vi "CCExcelToDcm.vi"(6 "DICOM Info":path, 8 "error in (no error)":errorcluster, 10 "JournalPath":path, 11 "ServerInfo":T1) -> (0 "error out":errorcluster, 1 "No active excel error":bool, 2 "VerificationFailure":string, 3 "FailureDescription":string)   [LabVIEW 2013, in "main.lvlib" / "ClearCanvasLibrary.lvlib"]
uses:
  ClearCanvasLibrary.lvlib
  C:/Users/Simon/SkyDrive/LabView/2013/DM2020/DICOM/ClearCanvasNewBuild/ClearCanvas.Dicom.dll
  ClearCanvasNewBuild/ClearCanvas.Dicom.dll
  <userlib>/_MGI/Error Handling/MGI Suppress Error Code/MGI Suppress Error Code (Scalar).vi
  main.lvlib
  Controls/Enum Variables.ctl
panel:
  in  "Excel._Worksheet":refnum<k7>
  in  "Excel._Application":refnum<k7>
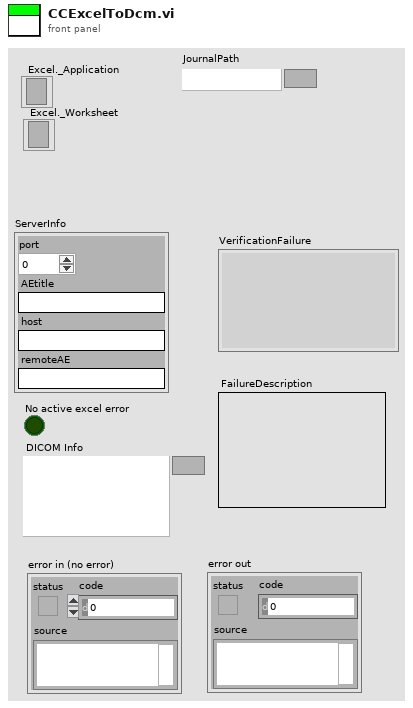
[diagram p1: front panel]
types:
  T1 = cluster{"port":i32, "AEtitle":string, "host":string, "remoteAE":string}
  T2 = typedef "main.lvlib/Enum Variables.ctl" = enum16{"SetAcqFilter", "GetAcqFilter", "Set Filter", "Get Filter", "Set Height", "Get Height", "Set Blue Pressure", "Get Blue Pressure", "Set Red Pressure", "Get Red Pressure", "Init", "Reset Pressure", "Set Red Cursors", "Get Red Cursors", "Set Blue Cursors", "Get Blue Cursors", "Set Language", "Get Language", "Set Active Graphs", "Get ActiveGraphs", "Set Method", "Get Method", "Set Encryption", "Get Encryption", "Set ExcelVersion", "Get ExcelVersion", "Set DICOM Avail", "Get DICOM Avail", "Set DICOM Encode", "Get DICOM Encode", "Set JournalExport", "Get JournalExport", "Set Sequence", "Get Sequence", "Set DAQ Connected", "Get DAQ Connected", "Set Current Graph", "Get Current Graph", "Set General Settings", "Get Hyphenation", "Set Arm Calc Method", "Get Arm Calc Method", "Set Dicom Tags", "Get Dicom Tags", "Set BT Serial", "Get BT Serial", "Set BT Accepted Serials", "Get BT Accepted Serials", "Get BT License", "Set BT License"}
  T3 = enum16{"leave excel open after last close", "close only if opened by LabVIEW", "close excel after last close"}
  T4 = enum16{"open workbook as template", "open workbook from file", "create new workbook"}
  T5 = typedef "excel Object Reference.ctl" = refnum<k1>
  T6 = typedef "excel Data Members.ctl" = cluster{"Excel._Application":refnum<k7>, "Excel._Workbook":refnum<k7>, "Excel._Worksheet":refnum<k7>, "template?":bool, "location":cluster{"TopLeft":string, "RightBottom":string}, "positioning info":cluster{"direction":enum16{"right", "down"}, "gap":i32}}
  T7 = cluster{"left":i16, "top":i16, "right":i16, "bottom":i16}
  T8 = cluster{"left":i32, "top":i32, "right":i32, "bottom":i32}
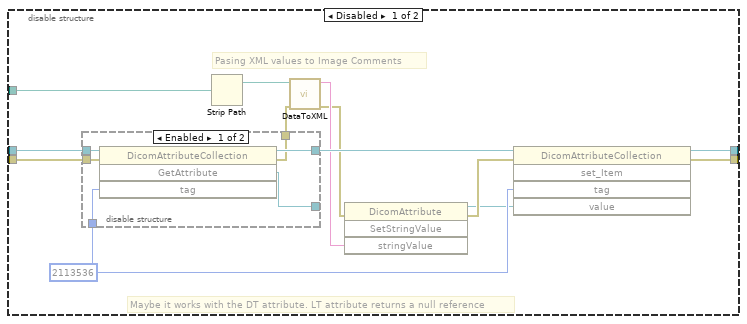
[diagram p2: hidden frame]
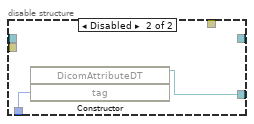
[diagram p3: hidden frame]
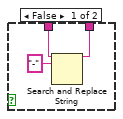
[diagram p4: hidden frame]
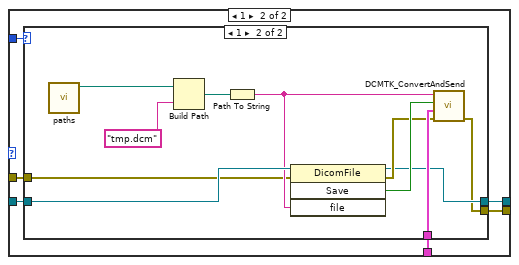
[diagram p5: hidden frame]
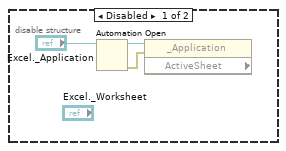
[diagram p7: hidden frame]
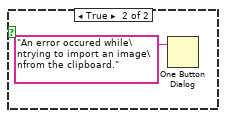
[diagram p8: hidden frame]
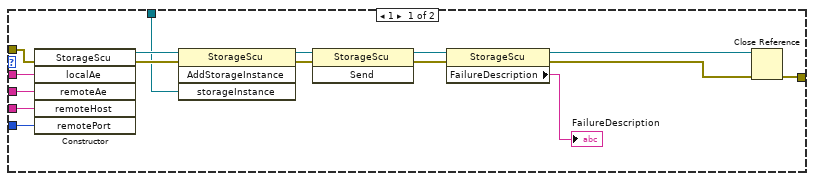
[diagram p9: hidden frame]
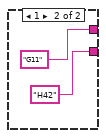
[diagram p11: hidden frame]
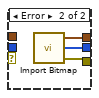
[diagram p12: hidden frame]
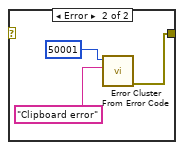
[diagram p13: hidden frame]
diagram:
  w67 = 6 items=["None", "CR", "CT", "MR", "NM", "US", "OT", "BI", "CD", "DD", "DG", "ES", "LS", "PT", "RG", "ST", "TG", "XA", "RF", "RTImage", "RTDose", "RTStruct", "RTPlan", "RTRecord", "HC", "DX", "MG", "IO", "PX", "GM", "SM", "XC", "PR", "AU", "Ecg", "Eps", "HD", "SR", "Ivus", "OP", "Smr", "Oct", "Opr", "Opv", "Opm", "KO", "Seg", "Reg", "DS", "CF", "DF", "VF", "AS", "CS", "EC", "LP", "FA", "CP", "DM", "FS", "MA", "MS"] ("Modality")
  n1 = disable-structure shown="Enabled" {
    frame Disabled {
      n2 = Automation Open(Automation Refnum="Excel._Application") -> (Automation Refnum=w150:refnum<k7>, error out=w149:errorcluster)  [unwired: 3 in]
      n3 = property class="_Application" props=["ActiveSheet"](reference=w150, error in=w149) -> ()  [unwired: 3 out]
    }
    frame Enabled {
    }
  }
  n4 = call <userlib>:"excel open (path).vi"("Visible (T)"=FALSE, "closing behavior (leave open)"=T3."close excel after last close", "worksheet_number"=u8 2, "workbook path"="JournalPath", "error in (no error)"="error in (no error)", "select/new"=enum16{"new sheet", "select sheet"}."select sheet", "create/open template/open file"=T4."open workbook from file") -> ("error out"=w31:errorcluster, "reference"=w32:T5)  [unwired: 3 in]
  n5 = call <userlib>:"excel Get Data to Modify.vi"("error in (no error)"=w31, "reference"=w32) -> ("error out"=w29:errorcluster, "data"=w23:T6, "duplicate reference"=w25:T5)  [unwired: 2 in, 1 out]
  n6 = Unbundle By Name(w23) -> ("Excel._Worksheet"=w30:refnum<k7>)
  n7 = while {
    tunnel: w29 -> [w165]
    tunnel: [w164] -> w96
    tunnel: [w159] -> w88
    tunnel: [w163] -> w92
    tunnel: [w160] -> w89
    tunnel: w30 -> [w155]
    stop <- w156 stop-if-true
    w169 = 2 items=["xlBitmap"=2, "xlPicture"=-4147] ("Format")
    w170 = 1 items=["xlPrinter"=2, "xlScreen"=1] ("Appearance")
    n8 = call "AE Variables.vi"("Action"=Enum_Variables."Get JournalExport") -> ("RingOut"=w152:u16)  [unwired: 11 in, 7 out]
    n9 = case shown="0, Default" w152 {
      tunnel: ["A1" "G11"] -> w168
      tunnel: ["H49" "H42"] -> w167
      frame 0, Default {
      }
      frame 1 {
      }
    }
    n10 = invoke class="_Worksheet" method="Range"(reference=w155, error in=w165, "Cell1"=w168, "Cell2"=w167) -> (error out=w166:errorcluster, "Range"=w171:refnum<k7>)  [unwired: 1 in, 3 out]
    n11 = invoke class="Range" method="CopyPicture"(reference=w171, error in=w166, "Appearance"=w170, "Format"=w169) -> (reference out=w160:refnum<k7>, error out=w154:errorcluster)  [unwired: 1 in, 3 out]
    n12 = case shown="No Error" w154 {
      selector: w154 -> [w176 w194]
      tunnel: [w182 _] -> w164
      tunnel: [w183 _] -> w163
      tunnel: [w180 w194] -> w159
      frame No Error {
        n13 = call "ImportBitmap2.vi"("error in (no error)"=w176) -> ("error out"=w177:errorcluster, "pixmap data"=w178:u8[], "rect"=w179:T7)  [unwired: 6 in, 2 out]
        n14 = case shown="No Error" w177 {
          selector: w177 -> [w184 _]
          tunnel: [w186 w189] -> w183
          tunnel: w179 -> [w186 _]
          tunnel: w178 -> [w185 _]
          tunnel: [w185 w188] -> w182
          tunnel: [w184 w187] -> w181
          frame No Error {
          }
          frame Error {
            n15 = call "Import Bitmap.vi"() -> ("rect"=w189:T8, "flattened data"=w188:u8[], "error out"=w187:errorcluster)  [unwired: 5 in, 2 out]
          }
        }
        n16 = case shown="No Error" w181 {
          selector: w181 -> [w190 _]
          tunnel: [w190 w193] -> w180
          frame No Error {
          }
          frame Error {
            n17 = call <vilib>:"Error Cluster From Error Code.vi"("error message (\"\")"="Clipboard error" ("error message (\"\")"), "error code (0)"=50001) -> ("error out"=w193:errorcluster)  [unwired: 7 in]
          }
        }
      }
      frame Error {
      }
    }
    n18 = Unbundle By Name(w159) -> ("status"=w157:bool)
    n19 = Unbundle By Name(w163) -> ("bottom"=w162:i32)
    n20 = Less?(x=500, y=w162) -> (x < y?=w158:bool)
    n21 = Or(x=w158, y=w157) -> (x .or. y?=w156:bool)
  }
  n22 = Close Reference(reference=w89, error in (no error)=w88) -> (error out=w28:errorcluster)
  n23 = Path To String(path="DICOM Info") -> (string=w18:string)
  n24 = call <userlib>:"excel Set Modified Data.vi"("error in (no error)"=w28, "data"=w23, "reference"=w25) -> ("error out"=w27:errorcluster, "duplicate reference"=w24:T5)  [unwired: 3 in]
  n25 = call <userlib>:"excel close.vi"("error in (no error)"=w27, "reference"=w24) -> ("error out"=w26:errorcluster)  [unwired: 9 in]
  n26 = invoke class="DicomUid" method="GenerateUid"(error in=w26) -> (error out=w147:errorcluster, "GenerateUid"=w102:refnum<k24>)  [unwired: 2 in, 1 out]
  n27 = constructor class="DicomTagDictionary"(error in=w26) -> (reference out=w141:refnum<k24>, error out=w137:errorcluster)  [unwired: 2 in, 1 out]
  n28 = constructor class="DicomFile"(error in=w26, "filename"=w18) -> (reference out=w101:refnum<k24>, error out=w100:errorcluster)  [unwired: 2 in, 2 out]
  n29 = invoke class="DicomFile" method="Load"(reference=w101, error in=w100) -> (reference out=w55:refnum<k24>, error out=w99:errorcluster)  [unwired: 1 in, 1 out]
  n30 = property class="DicomUid"(reference=w102, error in=w147) -> (reference out=w93:refnum<k24>, error out=w94:errorcluster, "UID"=w138:string)
  n31 = property class="DicomFile"(reference=w55, error in=w99, "MediaStorageSopClassUid"="1.2.840.10008.5.1.4.1.1.7" ("uid"), "MediaStorageSopInstanceUid"=w138, "TransferSyntaxUid"="1.2.840.10008.1.2.1") -> (reference out=w144:refnum<k24>, error out=w143:errorcluster)
  n32 = Close Reference(reference=w93, error in (no error)=w94) -> (error out=w9:errorcluster)
  n33 = invoke class="DicomTagDictionary" method="GetDicomTag"(reference=w141, error in=w137, "name"="SopInstanceUid") -> (reference out=w17:refnum<k24>, error out=w16:errorcluster, "GetDicomTag"=w139:refnum<k24>)  [unwired: 1 in, 1 out]
  n34 = property class="DicomFile"(reference=w144, error in=w143) -> (reference out=w54:refnum<k24>, error out=w107:errorcluster, "DataSet"=w142:refnum<k24>)
  n35 = constructor class="DicomAttributeUI"(error in=w107, "tag"=w139) -> (reference out=w130:refnum<k24>, error out=w132:errorcluster)  [unwired: 2 in, 2 out]
  n36 = invoke class="DicomAttributeUI" method="SetStringValue"(reference=w130, error in=w132, "stringValue"=w138) -> (reference out=w131:refnum<k24>, error out=w106:errorcluster)  [unwired: 1 in, 2 out]
  n37 = invoke class="DicomAttributeCollection" method="set_Item"(reference=w142, error in=w106, "tag"=w139, "value"=w131) -> (reference out=w2:refnum<k24>, error out=w1:errorcluster)  [unwired: 1 in, 3 out]
  n38 = disable-structure shown="Enabled" {
    disable-tunnel: "DICOM Info" -> [w207 _]
    disable-tunnel: [w206 w219] -> w11
    disable-tunnel: [w205 w218] -> w8
    disable-tunnel: w2 -> [w196 w219]
    disable-tunnel: w1 -> [w195 w218]
    frame Disabled {
      w204 = u32 2113536 ("tag")
      # "Pasing XML values to Image Comments"
      # "Maybe it works with the DT attribute. LT attribute returns a null reference"
      n39 = disable-structure shown="Enabled" {
        disable-tunnel: [w213 w216] -> w202
        disable-tunnel: [w212 w215] -> _
        disable-tunnel: [w211 w217] -> w198
        disable-tunnel: w204 -> [w210 w214]
        disable-tunnel: w196 -> [w209 _]
        disable-tunnel: w195 -> [w208 _]
        frame Enabled {
          n40 = invoke class="DicomAttributeCollection" method="GetAttribute"(reference=w209, error in=w208, "tag"=w210) -> (reference out=w213:refnum<k24>, error out=w211:errorcluster, "GetAttribute"=w212:refnum<k24>)  [unwired: 1 in, 1 out]
        }
        frame Disabled {
          n41 = constructor class="DicomAttributeDT"("tag"=w214) -> (reference out=w215:refnum<k24>)  [unwired: 3 in, 3 out]
        }
      }
      n42 = Strip Path(path=w207) -> (stripped path=w203:path)  [unwired: 1 out]
      n43 = call "DataToXML.vi"("error in"=w198, "path"=w203) -> ("error out"=w197:errorcluster, "XML"=w199:string)  [unwired: 8 in]
      n44 = invoke class="DicomAttribute" method="SetStringValue"(error in=w197, "stringValue"=w199) -> (reference out=w200:refnum<k24>, error out=w201:errorcluster)  [unwired: 2 in, 2 out]
      n45 = invoke class="DicomAttributeCollection" method="set_Item"(reference=w202, error in=w201, "tag"=w204, "value"=w200) -> (reference out=w206:refnum<k24>, error out=w205:errorcluster)  [unwired: 1 in, 3 out]
    }
    frame Enabled {
    }
  }
  n46 = invoke class="DicomTagDictionary" method="GetDicomTag"(reference=w17, error in=w16, "name"="SopClassUid") -> (reference out=w58:refnum<k24>, error out=w57:errorcluster, "GetDicomTag"=w109:refnum<k24>)  [unwired: 1 in, 1 out]
  n47 = Close Reference(reference=w58, error in (no error)=w57) -> (error out=w56:errorcluster)
  n48 = call "CCSetSpecificCharacterSet.vi"("error in (no error)"=w8, ".NET Refnum in"=w11) -> ("error out"=w7:errorcluster, ".NET Refnum out"=w10:refnum<k24>)  [unwired: 8 in]
  n49 = property class="SopClass"(error in=w56) -> (reference out=w61:refnum<k24>, error out=w60:errorcluster, "SecondaryCaptureImageStorageUid"=w111:string)  [unwired: 1 in]
  n50 = constructor class="DicomAttributeUI"(error in=w7, "tag"=w109) -> (reference out=w113:refnum<k24>, error out=w112:errorcluster)  [unwired: 2 in, 2 out]
  n51 = invoke class="DicomAttributeUI" method="SetStringValue"(reference=w113, error in=w112, "stringValue"=w111) -> (reference out=w110:refnum<k24>, error out=w108:errorcluster)  [unwired: 1 in, 2 out]
  n52 = Close Reference(reference=w61, error in (no error)=w60) -> (error out=w59:errorcluster)
  n53 = invoke class="DicomAttributeCollection" method="set_Item"(reference=w10, error in=w108, "tag"=w109, "value"=w110) -> (reference out=w5:refnum<k24>, error out=w91:errorcluster)  [unwired: 1 in, 3 out]
  n54 = Merge Errors(w91, w9, w59) -> (w90:errorcluster)
  n55 = constructor class="PatientModuleIod"(error in=w90, "dicomAttributeProvider"=w5) -> (reference out=w98:refnum<k24>, error out=w97:errorcluster)  [unwired: 2 in, 2 out]
  n56 = property class="PatientModuleIod"(reference=w98, error in=w97) -> (reference out=w73:refnum<k24>, error out=w72:errorcluster, "PatientsName"=w69:string, "PatientId"=w15:string)
  n57 = call "AE Variables.vi"("Action"=Enum_Variables."Get Hyphenation") -> ("BooleanOut"=w12:bool)  [unwired: 11 in, 7 out]
  n58 = case shown="True" w12 {
    tunnel: w15 -> [w222 w223]
    tunnel: [w220 w223] -> w14
    frame False {
      n59 = Search and Replace String(input string=w222, search string="-") -> (result string=w220:string)  [unwired: 6 in, 3 out]
    }
    frame True {
    }
  }
  n60 = call "NameToDICOMFormat.vi"("Name In"=w69) -> ("Name Out"=w68:string)  [unwired: 10 in]
  n61 = property class="PatientModuleIod"(reference=w73, error in=w72, "PatientsName"=w68, "PatientId"=w14) -> (reference out=w70:refnum<k24>, error out=w71:errorcluster)
  n62 = Close Reference(reference=w70, error in (no error)=w71) -> (error out=w127:errorcluster)
  n63 = constructor class="GeneralStudyModuleIod"(error in=w127, "dicomAttributeProvider"=w5) -> (reference out=w86:refnum<k24>, error out=w87:errorcluster)  [unwired: 2 in, 2 out]
  n64 = property class="GeneralStudyModuleIod"(reference=w86, error in=w87) -> (reference out=w85:refnum<k24>, error out=w84:errorcluster, "StudyInstanceUid"=w83:string, "ReferringPhysiciansName"=w75:string)
  n65 = call "CCExcelToDcmGenerateUIDs.vi"("String in"=w83) -> ("String out"=w82:string)  [unwired: 10 in]
  n66 = call "NameToDICOMFormat.vi"("Name In"=w75) -> ("Name Out"=w74:string)  [unwired: 10 in]
  n67 = property class="GeneralStudyModuleIod"(reference=w85, error in=w84, "StudyInstanceUid"=w82, "ReferringPhysiciansName"=w74) -> (reference out=w136:refnum<k24>, error out=w135:errorcluster)
  n68 = Close Reference(reference=w136, error in (no error)=w135) -> (error out=w129:errorcluster)
  n69 = constructor class="GeneralSeriesModuleIod"(error in=w129, "provider"=w5) -> (reference out=w81:refnum<k24>, error out=w80:errorcluster)  [unwired: 2 in, 2 out]
  n70 = property class="GeneralSeriesModuleIod"(reference=w81, error in=w80) -> (reference out=w79:refnum<k24>, error out=w78:errorcluster, "SeriesInstanceUid"=w77:string, "OperatorsName"=w66:string)
  n71 = call "NameToDICOMFormat.vi"("Name In"=w66) -> ("Name Out"=w65:string)  [unwired: 10 in]
  n72 = call "CCExcelToDcmGenerateUIDs.vi"("String in"=w77) -> ("String out"=w76:string)  [unwired: 10 in]
  n73 = property class="GeneralSeriesModuleIod"(reference=w79, error in=w78, "SeriesInstanceUid"=w76, "OperatorsName"=w65, "Modality"=w67) -> (reference out=w134:refnum<k24>, error out=w133:errorcluster)
  n74 = Close Reference(reference=w134, error in (no error)=w133) -> (error out=w128:errorcluster)
  n75 = constructor class="ImagePixelMacroIod"(error in=w128, "dicomAttributeProvider"=w5) -> (reference out=w126:refnum<k24>, error out=w64:errorcluster)  [unwired: 2 in, 2 out]
  n76 = property class="PhotometricInterpretation"(error in=w64) -> (error out=w63:errorcluster, "Rgb"=w115:refnum<k24>)  [unwired: 1 in, 1 out]
  n77 = invoke class="ImagePixelMacroIod" method="SetCommonTags"(reference=w126, error in=w63) -> (reference out=w125:refnum<k24>, error out=w124:errorcluster)  [unwired: 1 in, 1 out]
  n78 = Unbundle By Name(w92) -> ("right"=w117:i32, "bottom"=w116:i32)
  n79 = property class="ImagePixelMacroIod"(reference=w125, error in=w124, "BitsAllocated"=u16 8, "BitsStored"=u16 8, "HighBit"=u16 7, "PixelRepresentation"="0", "PlanarConfiguration"=u16 0, "SamplesPerPixel"=u16 3, "PixelData"=w96, "Columns"=w117, "Rows"=w116, "PhotometricInterpretation"=w115) -> (reference out=w62:refnum<k24>, error out=w95:errorcluster)
  n80 = Close Reference(reference=w62, error in (no error)=w95) -> (error out=w6:errorcluster)
  n81 = call "CCSetSpecificCharacterSet.vi"("error in (no error)"=w6, ".NET Refnum in"=w5) -> ("error out"=w3:errorcluster, ".NET Refnum out"=w4:refnum<k24>)  [unwired: 8 in]
  n82 = Close Reference(reference=w4, error in (no error)=w3) -> (error out=w48:errorcluster)
  n83 = Unbundle By Name("ServerInfo") -> ("AEtitle"=w45:string, "remoteAE"=w42:string, "host"=w43:string, "port"=w44:i32)
  n84 = call "CCVerificationSCU.vi"("remotePort"=w44, "error in (no error)"=w48, "remoteHost"=w43, "remoteAE"=w42, "clientAETitle"=w45) -> ("error out"=w47:errorcluster, "FailureDescription"=→"VerificationFailure":string, "Result"=w20:i32)  [unwired: 4 in]
  n85 = call "AE Variables.vi"("Action"=Enum_Variables."Get DICOM Encode") -> ("RingOut"=w51:u16)  [unwired: 11 in, 7 out]
  n86 = case shown="0, Default" w20 {
    tunnel: w54 -> [w224 w233]
    tunnel: [w224 w232] -> w53
    tunnel: w51 -> [_ w231]
    tunnel: [w225 w230] -> w50
    tunnel: w47 -> [w226 w229]
    tunnel: "ServerInfo" -> [_ w228]
    frame 0, Default {
      n87 = call <vilib>:"Error Cluster From Error Code.vi"("error in (no error)"=w226, "error code (0)"=51000) -> ("error out"=w225:errorcluster)  [unwired: 7 in]
    }
    frame 1 {
      n88 = case shown="1" w231 {
        tunnel: w233 -> [w235 w243]
        tunnel: w228 -> [_ w240]
        tunnel: w229 -> [w234 w239]
        tunnel: [w235 w237] -> w232
        tunnel: [w234 w236] -> w230
        frame 0, Default {
        }
        frame 1 {
          n89 = call "paths.vi"() -> ("PubAppData"=w246:path)  [unwired: 8 in, 3 out]
          n90 = Build Path(base path=w246, name or relative path="tmp.dcm") -> (appended path=w244:path)
          n91 = Path To String(path=w244) -> (string=w242:string)
          n92 = invoke class="DicomFile" method="Save"(reference=w243, error in=w239, "file"=w242) -> (reference out=w237:refnum<k24>, error out=w238:errorcluster, "Save"=w241:bool)  [unwired: 1 in, 1 out]
          n93 = call "DCMTK_ConvertAndSend.vi"("error in (no error)"=w238, "ServerInfo"=w240, "Saved?"=w241, "File Input"=w242) -> ("error out"=w236:errorcluster)  [unwired: 6 in, 1 out]
        }
      }
    }
  }
  n94 = case shown="0, Default" w51 {
    tunnel: [w257 w277] -> w146
    tunnel: w50 -> [w256 w277]
    tunnel: w53 -> [w255 _]
    tunnel: w45 -> [w251 _]
    tunnel: w42 -> [w250 _]
    tunnel: w43 -> [w249 _]
    tunnel: w44 -> [w248 _]
    tunnel: w20 -> [w247 _]
    frame 0, Default {
      n95 = constructor class="StorageInstance"(error in=w256, "dicomFile"=w255) -> (reference out=w254:refnum<k24>, error out=w252:errorcluster)  [unwired: 2 in, 2 out]
      n96 = case shown="0, Default" w247 {
        tunnel: [w265 w274] -> w253
        tunnel: w254 -> [w268 _]
        tunnel: w252 -> [w262 w275]
        tunnel: w251 -> [w261 _]
        tunnel: w250 -> [w260 _]
        tunnel: w249 -> [w259 _]
        tunnel: w248 -> [w258 _]
        frame 1 {
          n97 = constructor class="StorageScu"(error in=w262, "localAe"=w261, "remoteAe"=w260, "remoteHost"=w259, "remotePort"=w258) -> (reference out=w270:refnum<k24>, error out=w269:errorcluster)  [unwired: 2 in, 5 out]
          n98 = invoke class="StorageScu" method="AddStorageInstance"(reference=w270, error in=w269, "storageInstance"=w268) -> (reference out=w272:refnum<k24>, error out=w271:errorcluster)  [unwired: 1 in, 2 out]
          n99 = invoke class="StorageScu" method="Send"(reference=w272, error in=w271) -> (reference out=w264:refnum<k24>, error out=w263:errorcluster)  [unwired: 1 in, 1 out]
          n100 = property class="StorageScu"(reference=w264, error in=w263) -> (reference out=w267:refnum<k24>, error out=w266:errorcluster, "FailureDescription"=→"FailureDescription":string)
          n101 = Close Reference(reference=w267, error in (no error)=w266) -> (error out=w265:errorcluster)
        }
        frame 0, Default {
          n102 = call-poly <userlib>:"MGI Suppress Error Code.vi"("Error Code"=1172, "Error In"=w275) -> ("Error Out"=w274:errorcluster)  [unwired: 4 in, 1 out]
        }
      }
      n103 = Close Reference(reference=w254, error in (no error)=w253) -> (error out=w257:errorcluster)
    }
    frame 1 {
    }
  }
  n104 = Close Reference(reference=w53, error in (no error)=w146) -> (error out=w41:errorcluster)
  n105 = call-poly <userlib>:"MGI Suppress Error Code.vi"("Error Code"=50001, "Error In"=w41) -> ("Error Supressed?"=w39:bool, "Error Out"=w40:errorcluster)  [unwired: 4 in]
  n106 = case shown="False" w39 {
    frame False {
    }
    frame True {
      n107 = One Button Dialog(message="An error occured while\ntrying to import an image\nfrom the clipboard.") -> ()  [unwired: 1 in, 1 out]
    }
  }
  n108 = call-poly <userlib>:"MGI Suppress Error Code.vi"("Error Code"=97, "Error In"=w40) -> ("Error Supressed?"=→"No active excel error":bool, "Error Out"=→"error out":errorcluster)  [unwired: 4 in]
